vi "JSON To LVConstant Creator.vi"() -> ()   [LabVIEW 2018]
doc: "The wrapper engine to create a LabVIEW constant from JSON string."
uses:
  SLL Scripting/DataType/_Typedefs/Settings.ctl
  SLL Scripting/DataType/_Typedefs/Treat Null As.ctl
  <vilib>/numeric/LVNumericRepresentation.ctl
  <vilib>/Utility/error.llb/DialogType.ctl
  47753a47-97af-4612-b100-c4725a1216ea.vi
  <vilib>/JDP Science/JSONtext/JSON text to Variant.vi
  <vilib>/JDP Science/JSONtext/LVClass Serializer/JSONtext LVClass Serializer.lvclass
  SLL Scripting/SLL Scripting.lvlib
panel:
  in  "JSON":string="{\n     \"String\": \"Paste your JSON here\"\n}"
  in  "Settings":T1
  in  "Parse JSON":bool
  in  "Copy Constant":bool
  in  "Generate Constant":bool
  out "Logs":string
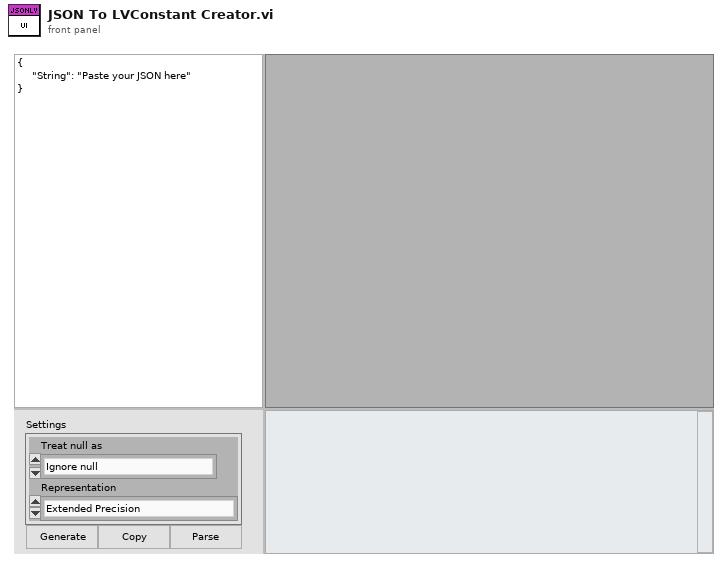
[diagram p1: front panel]
types:
  T1 = typedef "SLL Scripting.lvlib/Settings.ctl" = cluster{"Treat null as":T2, "Representation":T3}
  T2 = typedef "SLL Scripting.lvlib/Treat Null As.ctl" = enum16{"Ignore null", "Empty Object", "Empty Array", "String"}
  T3 = typedef "LVNumericRepresentation.ctl" = enum32{"Extended Precision", "Double Precision", "Single Precision", "Long", "Word", "Byte", "Unsigned Long", "Unsigned Word", "Unsigned Byte", "Complex Extended", "Complex Double", "Complex Single", "Quad", "Unsigned Quad", "Fixed-Point"}
  T4 = cluster{"JSON":string, "Log":string, "VI refnum":refnum<vi>, "owner refnum":refnum<vi>, "Settings":T1}
  T5 = typedef "DialogType.ctl" = u16
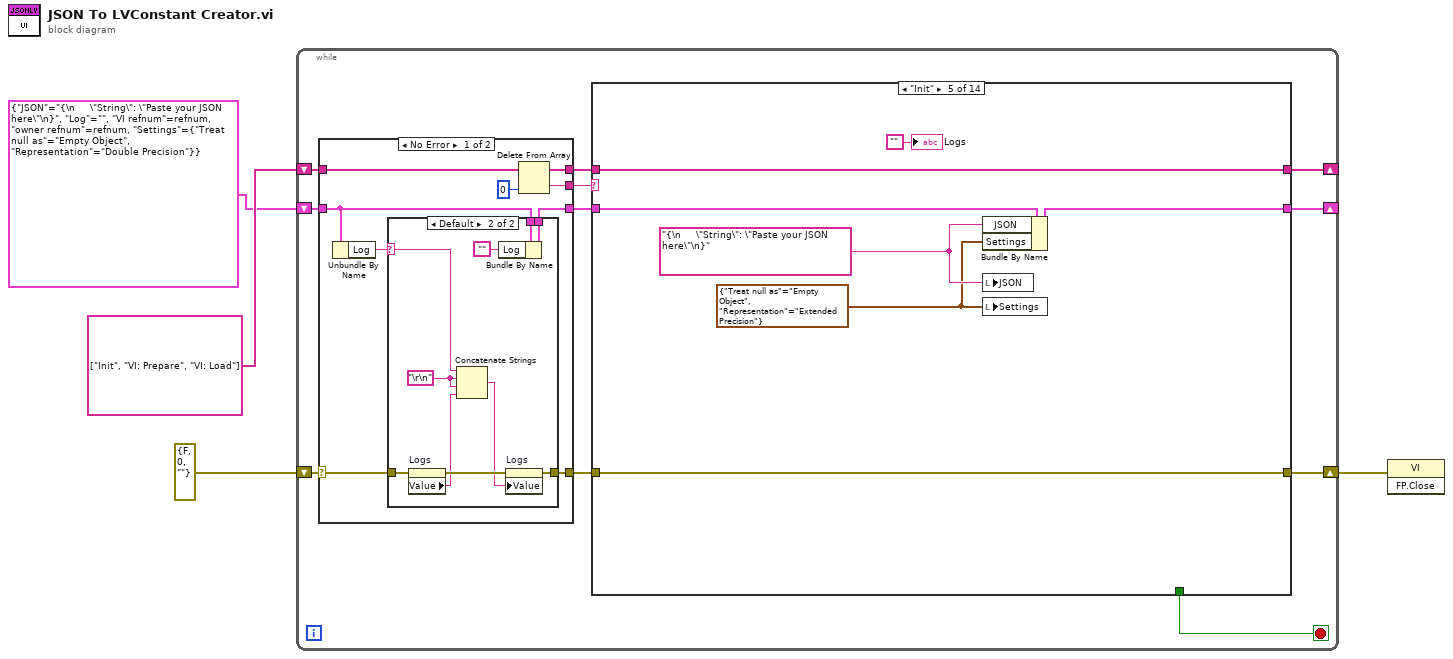
[diagram p0: block diagram]
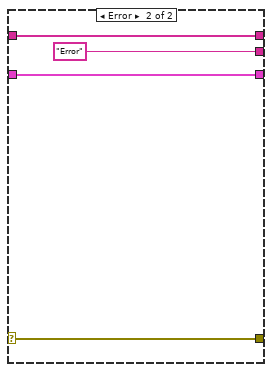
[diagram p3: hidden frame]
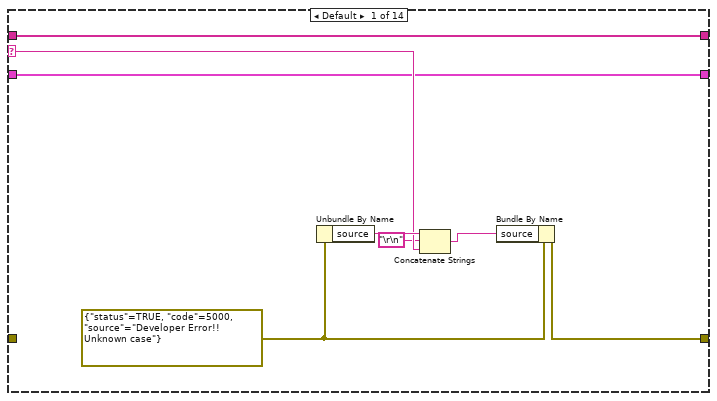
[diagram p4: hidden frame]
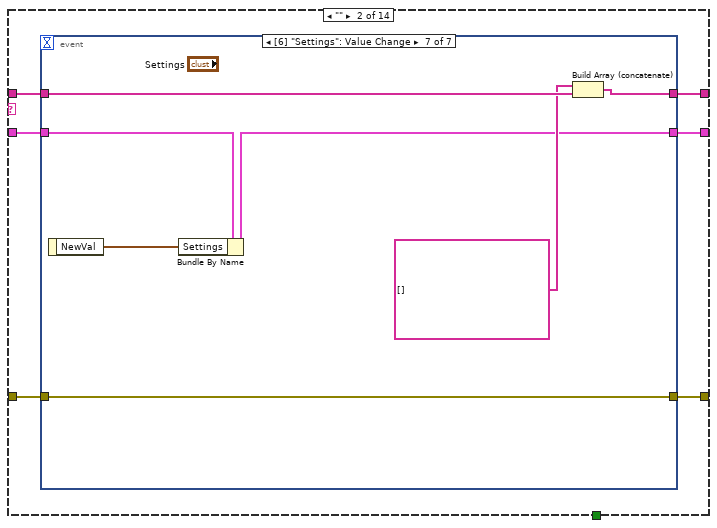
[diagram p5: hidden frame]
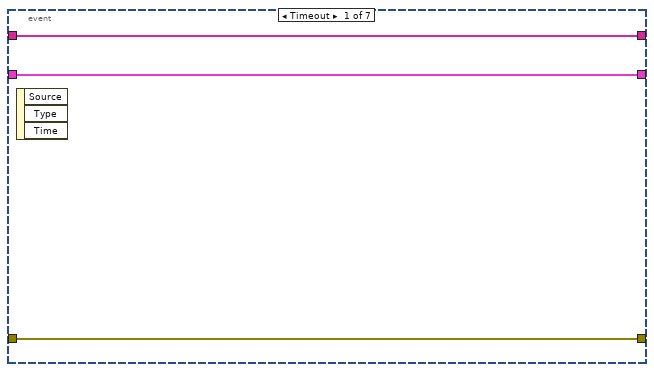
[diagram p6: hidden frame]
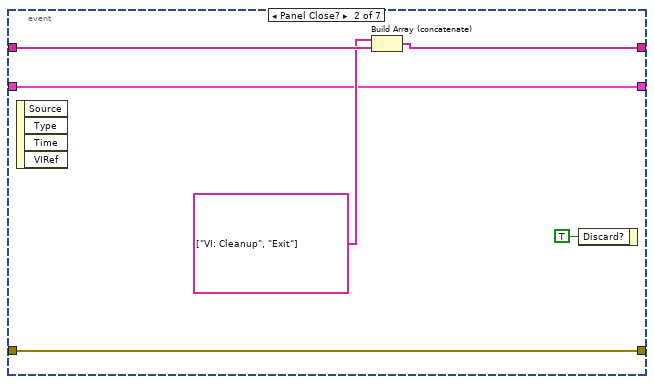
[diagram p7: hidden frame]
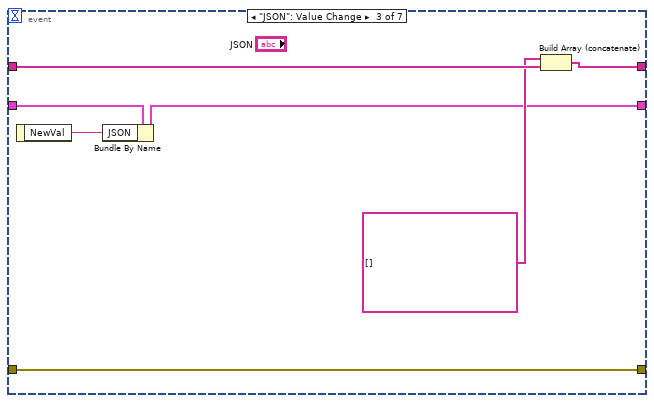
[diagram p8: hidden frame]
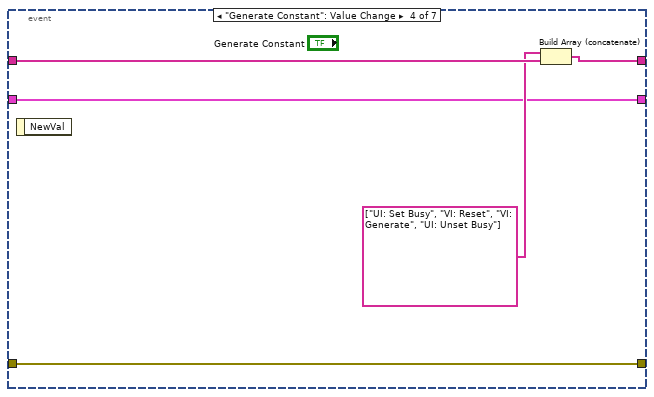
[diagram p9: hidden frame]
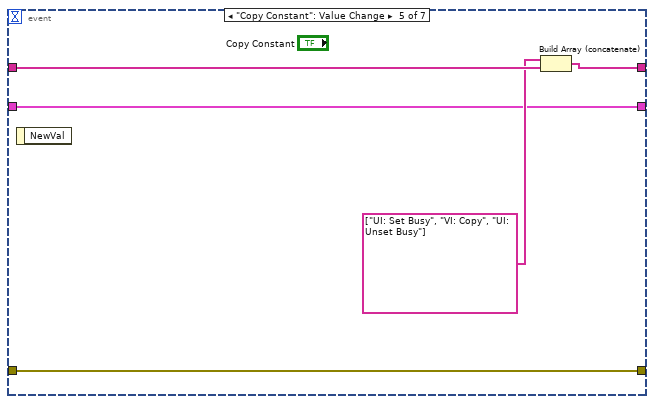
[diagram p10: hidden frame]
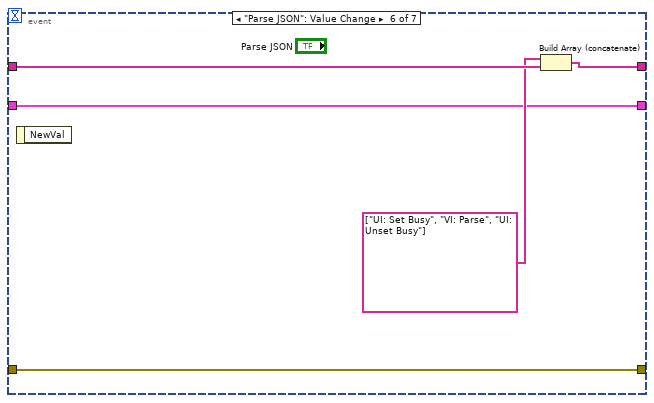
[diagram p11: hidden frame]
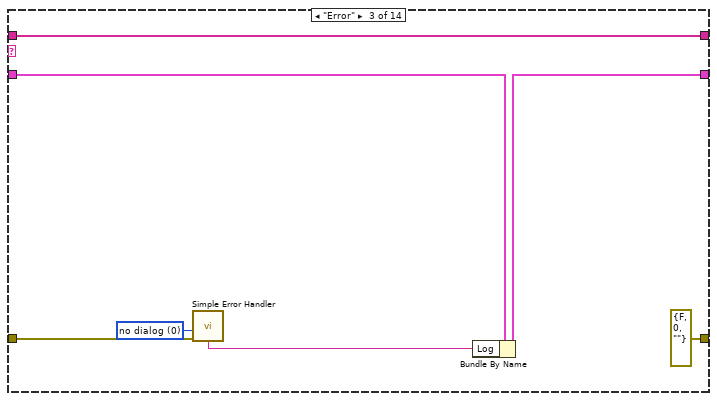
[diagram p12: hidden frame]
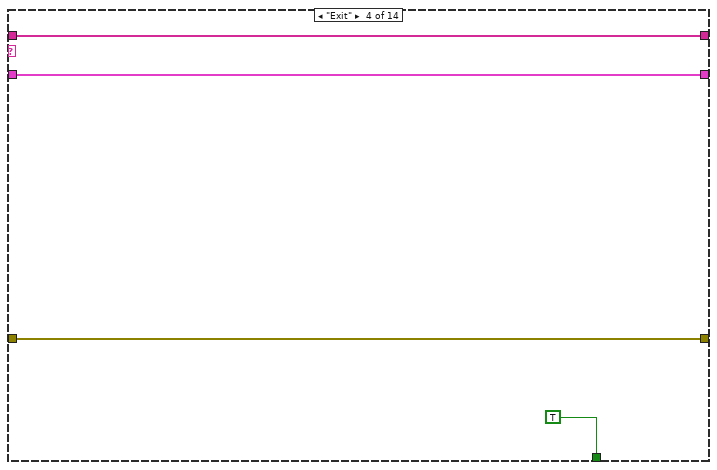
[diagram p13: hidden frame]
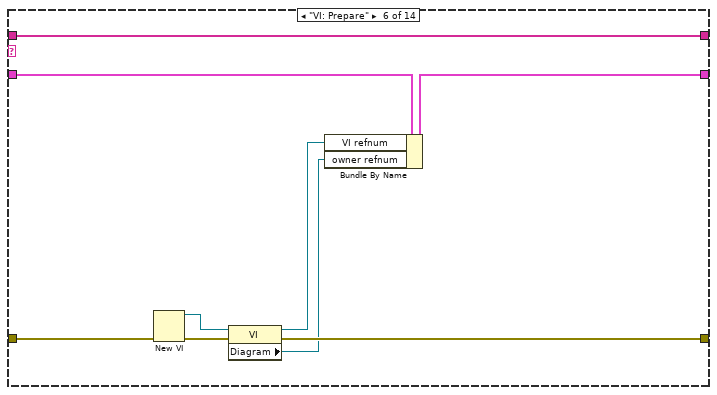
[diagram p14: hidden frame]
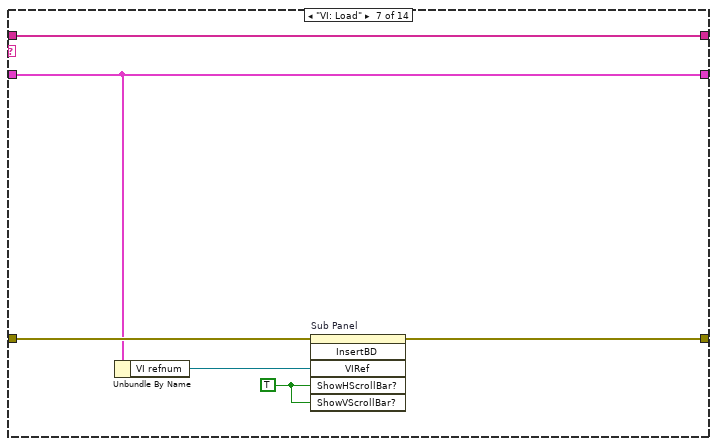
[diagram p15: hidden frame]
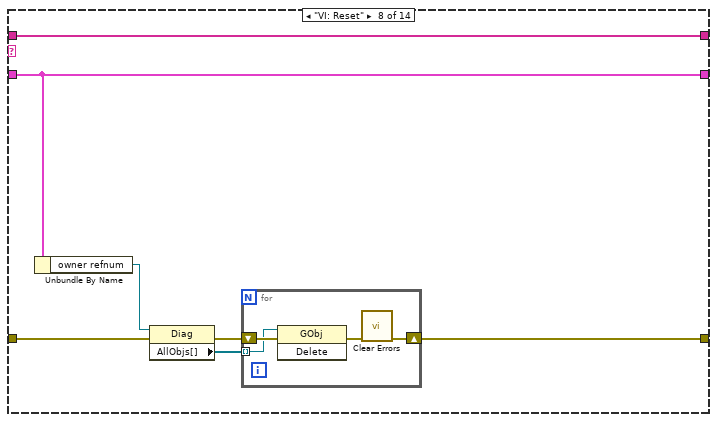
[diagram p16: hidden frame]
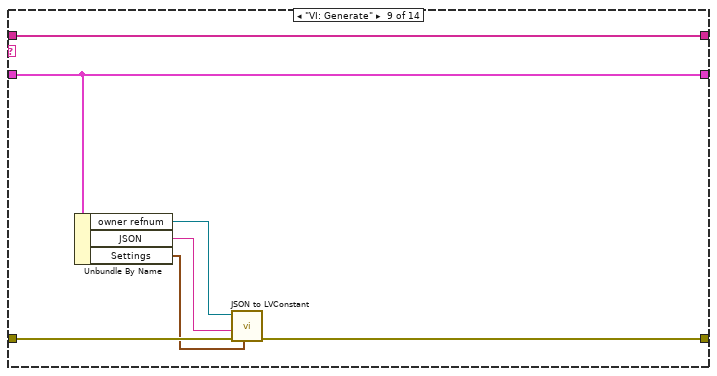
[diagram p17: hidden frame]
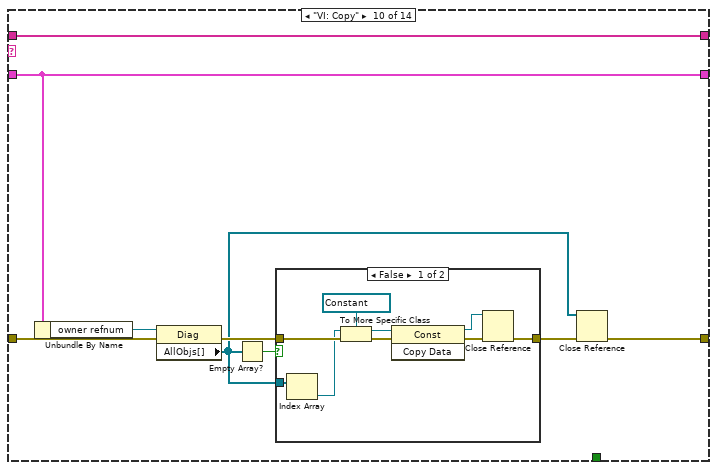
[diagram p18: hidden frame]
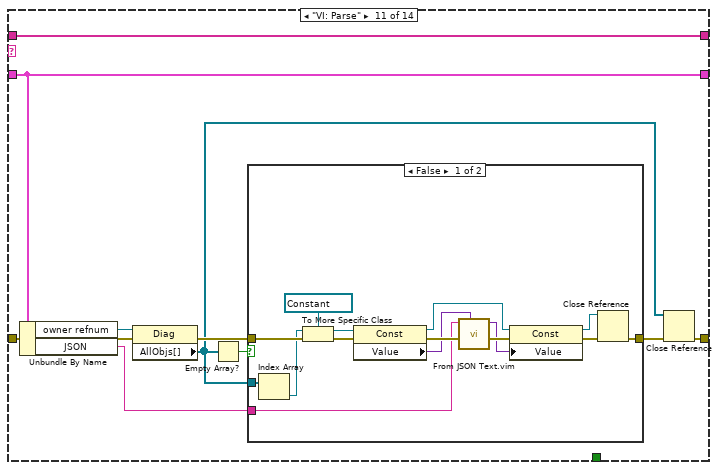
[diagram p20: hidden frame]
diagram:
  n1 = while {
    shift-right: [w15] -> w1
    shift-left: errorcluster {"status"=FALSE, "code"=0, "source"=""} ("error constant") -> [w13]
    shift-right: [w12] -> _
    shift-left: string[] ["Init", "VI: Prepare", "VI: Load"] -> [w10]
    shift-right: [w5] -> _
    shift-left: T4 {"JSON"="{\n     \"String\": \"Paste your JSON here\"\n}", "Log"="", "VI refnum"=refnum, "owner refnum"=refnum, "Settings"={"Treat null as"=enum."Empty Object", "Representation"=enum."Double Precision"}} -> [w6]
    stop <- w8 stop-if-true
    n2 = case shown="No Error" w13 {
      selector: w13 -> [w18 w38]
      tunnel: [w19 w38] -> w14
      tunnel: [w24 w40] -> w11
      tunnel: w10 -> [w23 w40]
      tunnel: [w21 "Error" ("String")] -> w9
      tunnel: [w16 w37] -> w7
      tunnel: w6 -> [w17 w37]
      frame No Error {
        n3 = Unbundle By Name(w17) -> ("Log"=w20:string)
        n4 = case shown="Default" w20 {
          selector: w20 -> [_ w31]
          tunnel: [w26 w34] -> w19
          tunnel: w18 -> [w26 w36]
          tunnel: w17 -> [w25 w29]
          tunnel: [w25 w28] -> w16
          frame "" {
          }
          frame Default {
            w30 = "\r\n"
            n5 = property on="Logs" class="Str"(error in=w36) -> (error out=w35:errorcluster, "Value"=w33:string)  [unwired: 1 in, 1 out]
            n6 = Concatenate Strings(w31, w30, w30, w33) -> (w32:string)
            n7 = Bundle By Name(cluster=w29, "Log"="") -> (w28:T4)
            n8 = property on="Logs" class="Str"(error in=w35, "Value"=w32) -> (error out=w34:errorcluster)  [unwired: 1 in, 1 out]
          }
        }
        n9 = Delete From Array(array=w23, index=0) -> (deleted portion=w21:string, array with subset deleted=w24:string[])  [unwired: 1 in]
      }
      frame Error {
      }
    }
    n10 = case shown="\"Init\"" w9 {
      selector: w9 -> [w43 _ _ _ _ _ _ _ _ _ _ _ _ _]
      tunnel: [w47 w54 errorcluster {"status"=FALSE, "code"=0, "source"=""} ("error IO") w103 w110 w115 w123 w128 w142 w146 w166 w194 w201 w212] -> w15
      tunnel: w14 -> [_ w53 w99 w103 w110 w116 w125 w132 w141 w152 w172 w197 w209 w220]
      tunnel: [w48 w52 w98 w102 w109 w119 w124 w131 w143 w151 w171 w198 w208 w219] -> w12
      tunnel: w11 -> [w48 w51 w98 w102 w109 w119 w124 w131 w143 w151 w171 w198 w208 w219]
      tunnel: [_ _ _ TRUE _ _ _ _ _ _ _ _ _ _] -> w8
      tunnel: w7 -> [w41 w49 w96 w100 w107 w118 w122 w130 w140 w150 w170 w196 w207 w218]
      tunnel: [w41 w50 w95 w100 w106 w113 w122 w130 w140 w150 w170 w196 w207 w218] -> w5
      frame Default {
        w46 = errorcluster {"status"=TRUE, "code"=5000, "source"="Developer Error!! Unknown case"} ("error constant")
        n11 = Unbundle By Name(w46) -> ("source"=w45:string)
        n12 = Concatenate Strings(w45, "\r\n", w43) -> (w44:string)
        n13 = Bundle By Name(cluster=w46, "source"=w44) -> (w47:errorcluster)
      }
      frame "" {
        n14 = event shown="[6] \"Settings\": Value Change" {
          selector: _ -> [_ _ _ _ _ _ _]
          dyn-events: _ -> [_ _ _ _ _ _ _]
          timeout: _ -> [_ _ _ _ _ _ _]
          tunnel: [w57 w63 w70 w75 w80 w85 w92] -> w54
          tunnel: w53 -> [w57 w63 w70 w75 w80 w85 w92]
          tunnel: [w56 w60 w68 w73 w78 w83 w90] -> w52
          tunnel: w51 -> [w56 w62 w69 w74 w79 w84 w91]
          tunnel: [w55 w58 w65 w71 w76 w81 w87] -> w50
          tunnel: w49 -> [w55 w58 w66 w71 w76 w81 w88]
          event Timeout {
            n15 = event-data() -> ()  [unwired: 1 in, 3 out]
          }
          event Panel Close? {
            n16 = event-data() -> ()  [unwired: 1 in, 4 out]
            n17 = Build Array (concatenate)(string[] ["VI: Cleanup", "Exit"], w62) -> (w60:string[])
            n18 = event-data("Discard?"=TRUE) -> ()  [unwired: 1 in, 1 out]
          }
          event "JSON": Value Change {
            n19 = event-data() -> ("NewVal"=w64:string)  [unwired: 1 in]
            n20 = Bundle By Name(cluster=w66, "JSON"=w64) -> (w65:T4)
            n21 = Build Array (concatenate)(string[] [], w69) -> (w68:string[])
          }
          event "Generate Constant": Value Change {
            n22 = event-data() -> ()  [unwired: 1 in, 1 out]
            n23 = Build Array (concatenate)(string[] ["UI: Set Busy", "VI: Reset", "VI: Generate", "UI: Unset Busy"], w74) -> (w73:string[])
          }
          event "Copy Constant": Value Change {
            n24 = event-data() -> ()  [unwired: 1 in, 1 out]
            n25 = Build Array (concatenate)(string[] ["UI: Set Busy", "VI: Copy", "UI: Unset Busy"], w79) -> (w78:string[])
          }
          event "Parse JSON": Value Change {
            n26 = event-data() -> ()  [unwired: 1 in, 1 out]
            n27 = Build Array (concatenate)(string[] ["UI: Set Busy", "VI: Parse", "UI: Unset Busy"], w84) -> (w83:string[])
          }
          event Value Change {
            n28 = event-data() -> ("NewVal"=w86:T1)  [unwired: 1 in]
            n29 = Bundle By Name(cluster=w88, "Settings"=w86) -> (w87:T4)
            n30 = Build Array (concatenate)(string[] [], w91) -> (w90:string[])
          }
        }
      }
      frame "Error" {
        w97 = T5 0 items=["no dialog", "OK message", "continue or stop message", "OK message + warnings", "continue/stop + warnings"] ("type of dialog (OK msg:1)")
        n31 = call <vilib>:"Simple Error Handler.vi"("type of dialog (OK msg:1)"=w97, "error in (no error)"=w99) -> ("message"=w94:string)  [unwired: 3 in, 4 out]
        n32 = Bundle By Name(cluster=w96, "Log"=w94) -> (w95:T4)
      }
      frame "Exit" {
      }
      frame "Init" {
        w104 = T1 {"Treat null as"=enum."Empty Object", "Representation"=enum."Extended Precision"} ("Settings")
        w105 = "{\n     \"String\": \"Paste your JSON here\"\n}" ("JSON")
        n33 = Bundle By Name(cluster=w107, "JSON"=w105, "Settings"=w104) -> (w106:T4)
        n34 = local write "JSON"(w105) -> ()
        n35 = local write "Settings"(w104) -> ()
        "Logs" <- "" ("Logs")
      }
      frame "VI: Prepare" {
        n36 = New VI(8:w116) -> (0:w117:errorcluster, 3:w114:refnum<vi>)  [unwired: 6 in]
        n37 = property class="VI"(reference=w114, error in=w117) -> (reference out=w112:refnum<vi>, error out=w115:errorcluster, "Diagram"=w111:refnum<vi>)
        n38 = Bundle By Name(cluster=w118, "VI refnum"=w112, "owner refnum"=w111) -> (w113:T4)
      }
      frame "VI: Load" {
        w120 = TRUE ("ShowHScrollBar")
        n39 = Unbundle By Name(w122) -> ("VI refnum"=w121:refnum<vi>)
        n40 = invoke on="Sub Panel" class="SubPnl" method="InsertBD"(error in=w125, "VIRef"=w121, "ShowHScrollBar?"=w120, "ShowVScrollBar?"=w120) -> (error out=w123:errorcluster)  [unwired: 2 in, 5 out]
      }
      frame "VI: Reset" {
        n41 = Unbundle By Name(w130) -> ("owner refnum"=w129:refnum<vi>)
        n42 = property class="Diag"(reference=w129, error in=w132) -> (error out=w127:errorcluster, "AllObjs[]"=w126:refnum<vi>[])  [unwired: 1 out]
        n43 = for {
          shift-right: [w133] -> w128
          shift-left: w127 -> [w136]
          tunnel: w126 -> [w134] mode=indexing
          n44 = invoke class="GObj" method="Delete"(reference=w134, error in=w136) -> (error out=w135:errorcluster)  [unwired: 1 in, 2 out]
          n45 = call <vilib>:"Clear Errors.vi"("error in (no error)"=w135) -> ("error out"=w133:errorcluster)  [unwired: 5 in, 1 out]
        }
      }
      frame "VI: Generate" {
        n46 = Unbundle By Name(w140) -> ("owner refnum"=w139:refnum<vi>, "JSON"=w138:string, "Settings"=w137:T1)
        n47 = call "JSON to LVConstant.vi"("Settings"=w137, "error in (no error)"=w141, "<JSON>"=w138, "owner refnum in"=w139) -> ("error out"=w142:errorcluster)  [unwired: 6 in, 1 out]
      }
      frame "VI: Copy" {
        n48 = Unbundle By Name(w150) -> ("owner refnum"=w149:refnum<vi>)
        n49 = property class="Diag"(reference=w149, error in=w152) -> (error out=w148:errorcluster, "AllObjs[]"=w144:refnum<vi>[])  [unwired: 1 out]
        n50 = Empty Array?(array=w144) -> (empty?=w145:bool)
        n51 = case shown="False" w145 {
          tunnel: w148 -> [w161 w162]
          tunnel: [w155 w162] -> w147
          tunnel: w144 -> [w153 _]
          frame False {
            n52 = Index Array(array=w153) -> (element=w158:refnum<vi>)  [unwired: 1 in]
            n53 = To More Specific Class(target class=refnum<vi> refnum ("reference"), reference=w158, error in=w161) -> (specific class reference=w157:refnum<vi>, error out=w159:errorcluster)
            n54 = invoke class="Const" method="Copy Data"(reference=w157, error in=w159) -> (reference out=w154:refnum<vi>, error out=w160:errorcluster)  [unwired: 1 in, 1 out]
            n55 = Close Reference(reference=w154, error in (no error)=w160) -> (error out=w155:errorcluster)
          }
          frame True {
          }
        }
        n56 = Close Reference(reference=w144, error in (no error)=w147) -> (error out=w146:errorcluster)
      }
      frame "VI: Parse" {
        n57 = Unbundle By Name(w170) -> ("owner refnum"=w169:refnum<vi>, "JSON"=w163:string)
        n58 = property class="Diag"(reference=w169, error in=w172) -> (error out=w168:errorcluster, "AllObjs[]"=w164:refnum<vi>[])  [unwired: 1 out]
        n59 = Empty Array?(array=w164) -> (empty?=w165:bool)
        n60 = case shown="False" w165 {
          tunnel: w168 -> [w187 w188]
          tunnel: [w181 w188] -> w167
          tunnel: w164 -> [w180 _]
          tunnel: w163 -> [w178 _]
          frame False {
            n61 = Index Array(array=w180) -> (element=w184:refnum<vi>)  [unwired: 1 in]
            n62 = To More Specific Class(target class=refnum<vi> refnum ("reference"), reference=w184, error in=w187) -> (specific class reference=w183:refnum<vi>, error out=w185:errorcluster)
            n63 = property class="Const"(reference=w183, error in=w185) -> (reference out=w175:refnum<vi>, error out=w186:errorcluster, "Value"=w177:variant)
            n64 = call "From JSON Text.vim"("Data Type and Default Value"=w177, "error in (no error)"=w186, "JSON"=w178) -> ("error out"=w179:errorcluster, "Data out"=w173:variant)  [unwired: 7 in]
            n65 = property class="Const"(reference=w175, error in=w179, "Value"=w173) -> (reference out=w174:refnum<vi>, error out=w176:errorcluster)
            n66 = Close Reference(reference=w174, error in (no error)=w176) -> (error out=w181:errorcluster)
          }
          frame True {
          }
        }
        n67 = Close Reference(reference=w164, error in (no error)=w167) -> (error out=w166:errorcluster)
      }
      frame "VI: Cleanup" {
        n68 = Unbundle By Name(w196) -> ("VI refnum"=w191:refnum<vi>, "owner refnum"=w193:refnum<vi>)
        n69 = Close Reference(reference=w193, error in (no error)=w197) -> (error out=w195:errorcluster)
        n70 = invoke class="VI" method="FP.Close"(reference=w191, error in=w195) -> (reference out=w190:refnum<vi>, error out=w192:errorcluster)  [unwired: 1 in, 1 out]
        n71 = call <vilib>:"Clear Errors.vi"("error in (no error)"=w192) -> ("error out"=w189:errorcluster)  [unwired: 5 in, 1 out]
        n72 = Close Reference(reference=w190, error in (no error)=w189) -> (error out=w194:errorcluster)
      }
      frame "UI: Set Busy" {
        n73 = Unbundle By Name(w207) -> ("VI refnum"=w205:refnum<vi>)
        n74 = property class="VI"(reference=w205, error in=w209) -> (error out=w206:errorcluster, "Panel"=w203:refnum<vi>)  [unwired: 1 out]
        n75 = property class="Pnl"(reference=w203, error in=w206, "DeferPanUpdts"=TRUE ("Defer Panel Updates")) -> (reference out=w199:refnum<vi>, error out=w204:errorcluster)
        n76 = Close Reference(reference=w199, error in (no error)=w204) -> (error out=w200:errorcluster)
        n77 = call <vilib>:"Set Busy.vi"("error in (no error)"=w200) -> ("error out"=w201:errorcluster)  [unwired: 9 in, 1 out]
      }
      frame "UI: Unset Busy" {
        n78 = Unbundle By Name(w218) -> ("VI refnum"=w216:refnum<vi>)
        n79 = property class="VI"(reference=w216, error in=w220) -> (error out=w217:errorcluster, "Panel"=w214:refnum<vi>)  [unwired: 1 out]
        n80 = property class="Pnl"(reference=w214, error in=w217, "DeferPanUpdts"=FALSE ("Defer Panel Updates")) -> (reference out=w210:refnum<vi>, error out=w215:errorcluster)
        n81 = Close Reference(reference=w210, error in (no error)=w215) -> (error out=w211:errorcluster)
        n82 = call <vilib>:"Unset Busy.vi"("error in (no error)"=w211) -> ("error out"=w212:errorcluster)  [unwired: 10 in]
      }
    }
  }
  n83 = invoke class="VI" method="FP.Close"(error in=w1) -> ()  [unwired: 2 in, 3 out]
